vi "New Data.vi"(6 "dt":dbl, 8 "error in (no error)":errorcluster, 9 "t0":dbl, 10 "Data":dbl[][](array[numeric]), 11 "DataHandlerAPI in":refnum<class "DataHandlerAPI.lvclass">) -> (0 "error out":errorcluster, 3 "DataHandlerAPI out":refnum<class "DataHandlerAPI.lvclass">)   [LabVIEW 2020, in "Volatus.lvlib" / "DataHandlerAPI.lvclass"]
uses:
  DataHandlerAPI.lvclass
  DataHandlerAPI.lvclass/DataHandlerAPI.ctl
  DataHandler Messages/New Data Msg/New Data Msg.lvclass
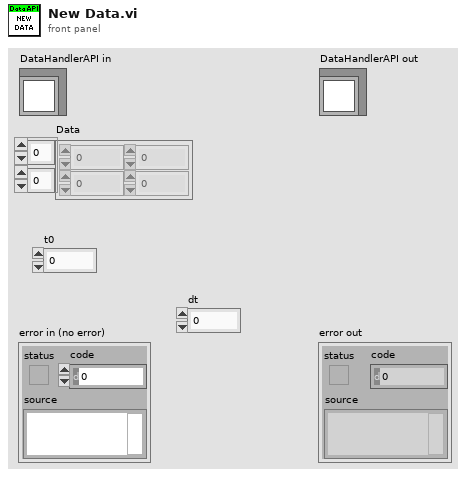
[diagram p1: front panel]
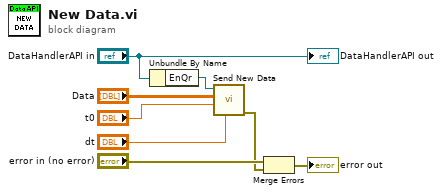
[diagram p0: block diagram]
diagram:
  n1 = Unbundle By Name("DataHandlerAPI in") -> ("EnQr"=w6:refnum<class "Message Enqueuer.lvclass">)
  n2 = call "Send New Data.vi"("dt"="dt", "t0"="t0", "Data"="Data", "Message Enqueuer"=w6) -> ("error out"=w1:errorcluster)  [unwired: 6 in, 1 out]
  n3 = Merge Errors("error in (no error)", w1) -> (→"error out":errorcluster)
  "DataHandlerAPI out" <- "DataHandlerAPI in"
